vi "SendDutyCycleProtocol.vi"(7 "Send":bool, 9 "Initialize":bool, 10 "Previous":T1={"type"="AI", "device"="", "name"="", "data"={"<init"=FALSE, ">position"=0.0, ">connected"=FALSE}}, 11 "Current":T1={"type"="AI", "device"="", "name"="", "data"={"<init"=FALSE, ">position"=0.0, ">connected"=FALSE}}) -> ()   [LabVIEW 2019]
uses:
  DutyCycle proto.ctl
  DutyCycle Data proto.ctl
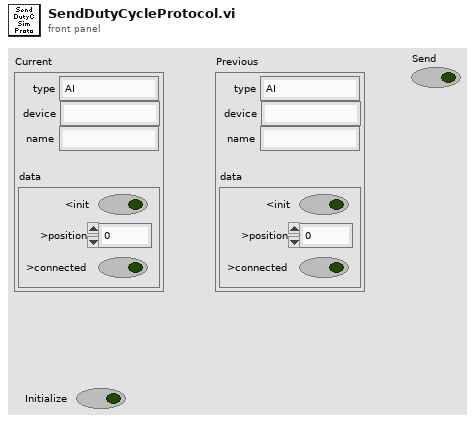
[diagram p1: front panel]
types:
  T1 = typedef "DutyCycle proto.ctl" = cluster{"type":string, "device":string, "name":string, "data":T2}
  T2 = typedef "DutyCycle Data proto.ctl" = cluster{"<init":bool, ">position":dbl, ">connected":bool}
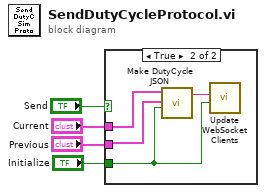
[diagram p0: block diagram]
diagram:
  n1 = case shown="True" "Send" {
    tunnel: "Current" -> [_ w8]
    tunnel: "Previous" -> [_ w7]
    tunnel: "Initialize" -> [_ w6]
    frame False {
    }
    frame True {
      n2 = call "Make DutyCycle JSON.vi"("Force"=w6, "Previous"=w7, "New"=w8) -> ("delta JSON"=w5:string)  [unwired: 8 in]
      n3 = call "Update WebSocket Clients.vi"("Initialize"=w6, "delta JSON"=w5) -> ()  [unwired: 10 in]
    }
  }
